vi "IOS_Ephys_WhiskerTracking_Master.vi"() -> ()   [LabVIEW 2013]
uses:
  <vilib>/userdefined/High Color/IMAQdx.ctl
  <vilib>/vision/driver/IMAQdx.llb/IMAQdx Acquisition Mode.ctl
  <vilib>/vision/driver/IMAQdx.llb/IMAQdx Camera Control Mode.ctl
  <vilib>/vision/driver/IMAQdx.llb/IMAQdx Buffer Number Mode.ctl
  <vilib>/DAQmx/read.llb/DAQmx Read (Analog 1D Wfm NChan NSamp).vi
  <vilib>/DAQmx/write.llb/DAQmx Write (Digital 1D Bool NChan 1Samp 1Line).vi
  <vilib>/DAQmx/create/channels.llb/DAQmx Create Channel (DO-Digital Output).vi
  <vilib>/DAQmx/create/channels.llb/DAQmx Create Channel (CO-Pulse Generation-Frequency).vi
  <vilib>/DAQmx/configure/timing.llb/DAQmx Timing (Implicit).vi
  <vilib>/DAQmx/create/channels.llb/DAQmx Create Channel (AI-Voltage-Basic).vi
  <vilib>/DAQmx/configure/timing.llb/DAQmx Timing (Sample Clock).vi
  <vilib>/DAQmx/configure/trigger.llb/DAQmx Start Trigger (Digital Edge).vi
  <vilib>/DAQmx/miscellaneous.llb/DAQmx Fill In Error Info.vi
  <vilib>/vision/driver/NI_Vision_Acquisition_Software.lvlib
panel:
  in  "physical channels":tag="Dev1/ai0:5"
  in  "Whisker Cam ID":T1="cam2"
  in  "WebCam ID":T1="cam1"
  in  "Analog Acquisition Setup":cluster{"Analog Sampling Rate":u16}={"Analog Sampling Rate"=20000} {"Analog Sampling Rate" format="%0.0f"}
  in  "Camera Acquisition Setup":T2={"CBVCam Rate"=30, "WhiskerCam Rate"=150, "WebCam Rate"=15}
  out "Notes Size":i32=7
  out "Notes Reversed":string[](array[string])=["Experimenter", "Animal ID", "Imaged Hemisphere", "Solenoid Pressure", "Isoflurane time", "Session ID", "Amplifier Gain"]
  out "Notes Array":string[](array[string])=["Amplifier Gain", "Session ID", "Isoflurane time", "Solenoid Pressure", "Imaged Hemisphere", "Animal ID", "Experimenter"]
  in  "Session Notes:":T3={"Experimenter"="Experimenter", "Animal ID"="ID", "Imaged Hemisphere"="Hem", "Solenoid Pressure"="psi", "Isoflurane time"="0000", "Session ID"="Test", "Amplifier Gain"="10000"}
  in  "Whisker Cam\nTrigger Source":tag="Dev1/ctr1"
  in  "CBV Cam\nTrigger Source":tag="Dev1/ctr0"
  in  "Left Pad":tag="Dev1/port0/line1"
  in  "Right Pad":tag="Dev1/port0/line0"
  in  "Ctl":tag="Dev1/port0/line3"
  in  "Tail":tag="Dev1/port0/line2"
  in  "Stim \nOffset (s)":dbl=30.0
  in  "Stim \nDuration (s)":dbl=0.1 step=0.1
  in  "Inter-Stim\nInterval (s)":dbl=60.0
  in  "Left Pad":dbl=1.0
  in  "Right Pad":dbl=1.0
  in  "Ctl":dbl=1.0
  in  "Tail":dbl=1.0
  in  "Target Path":path=path "D:/LabVIEW Test Data" caption="Final Saved Location for Files"
  out "Dropped":u32(slide) caption="Dropped Whisker\nCamera Frames" scale=0.0..50.0
  out "Analog file name":string="170302_16_55_2302"
  out "Actual WebCam Frame Rate":dbl(knob)=53292.6 scale=0.0..30.0
  out "WebCam":T4(plugin-control)
  out "Finished Acquiring":bool
  out "Trial Time Elapsed (Min)":cluster{dbl, dbl}(slide)={5.0, 0.09035140000000001} scale=0.0..5.0
  in  "Recording Time (min)":dbl(knob)=5.0 min=0.5 max=10.0 step=0.5 scale=0.0..5.0 scale format="%#_2g"
  in  "Temp Path":path=path "C:/LabView Test Files" caption="Temporary Path for Streamed Data"
  out "Last CBV\nBuffer":i32=162
  in  "Stop":bool
  out "Actual CBVCam\nFrame Rate":dbl(knob)=30.0 scale=0.0..60.0
  out "Last Whisk\nBuffer":u32
  out "Actual WhiskCam\nFrame Rate":dbl(knob) scale=0.0..300.0
  # "File Settings:"
  # "Stimulation Settings:"
  # "Stim. Ratios:"
  # "Output Channels:"
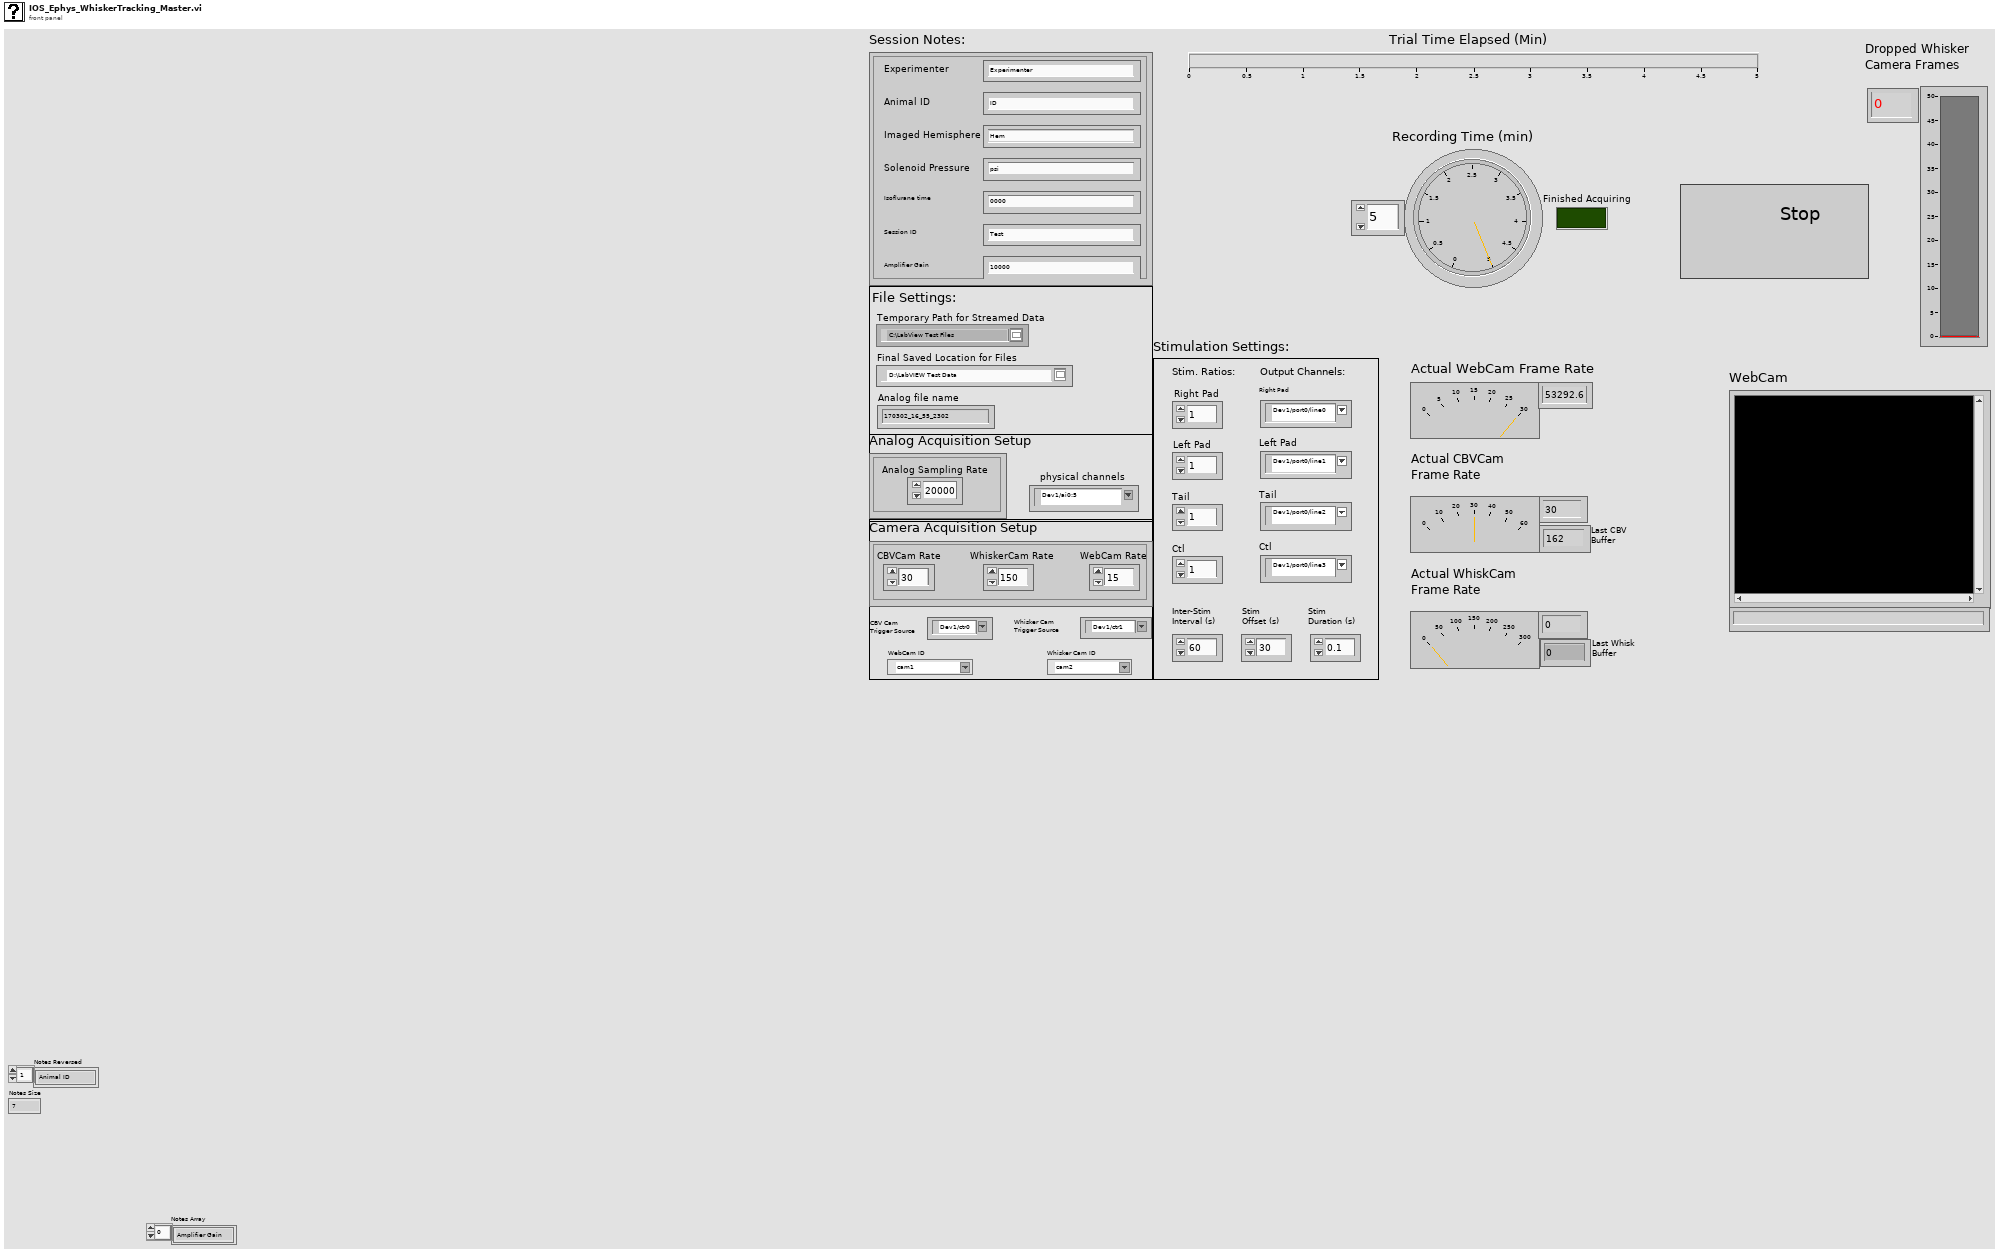
[diagram p1: front panel]
types:
  T1 = typedef "IMAQdx.ctl" = refnum<k21>
  T2 = cluster{"CBVCam Rate":u16, "WhiskerCam Rate":u16, "WebCam Rate":u16}
  T3 = cluster{"Experimenter":string, "Animal ID":string, "Imaged Hemisphere":string, "Solenoid Pressure":string, "Isoflurane time":string, "Session ID":string, "Amplifier Gain":string}
  T4 = typedef "IMAQ Image.ctl" = refnum<image>
  T5 = enum16{"open", "open or create", "create or replace", "create", "open (read-only)"}
  T6 = typedef "Image Type" = u32
  T7 = typedef "NI_Vision_Acquisition_Software.lvlib/IMAQdx Camera Control Mode.ctl" = enum32{"Controller", "Listener"}
  T8 = enum16{"open", "replace", "create", "open or create", "replace or create", "replace or create with confirmation"}
  T9 = typedef "NI_Vision_Acquisition_Software.lvlib/IMAQdx Acquisition Mode.ctl" = enum32{"One Shot", "Continuous"}
  T10 = typedef "IMAQ AVI2 Refnum.ctl" = refnum<k20>
  T11 = enum16{"big-endian, network order", "native, host order", "little-endian"}
  T12 = typedef "NI_Vision_Acquisition_Software.lvlib/IMAQdx Buffer Number Mode.ctl" = enum32{"Next", "Last", "Buffer Number"}
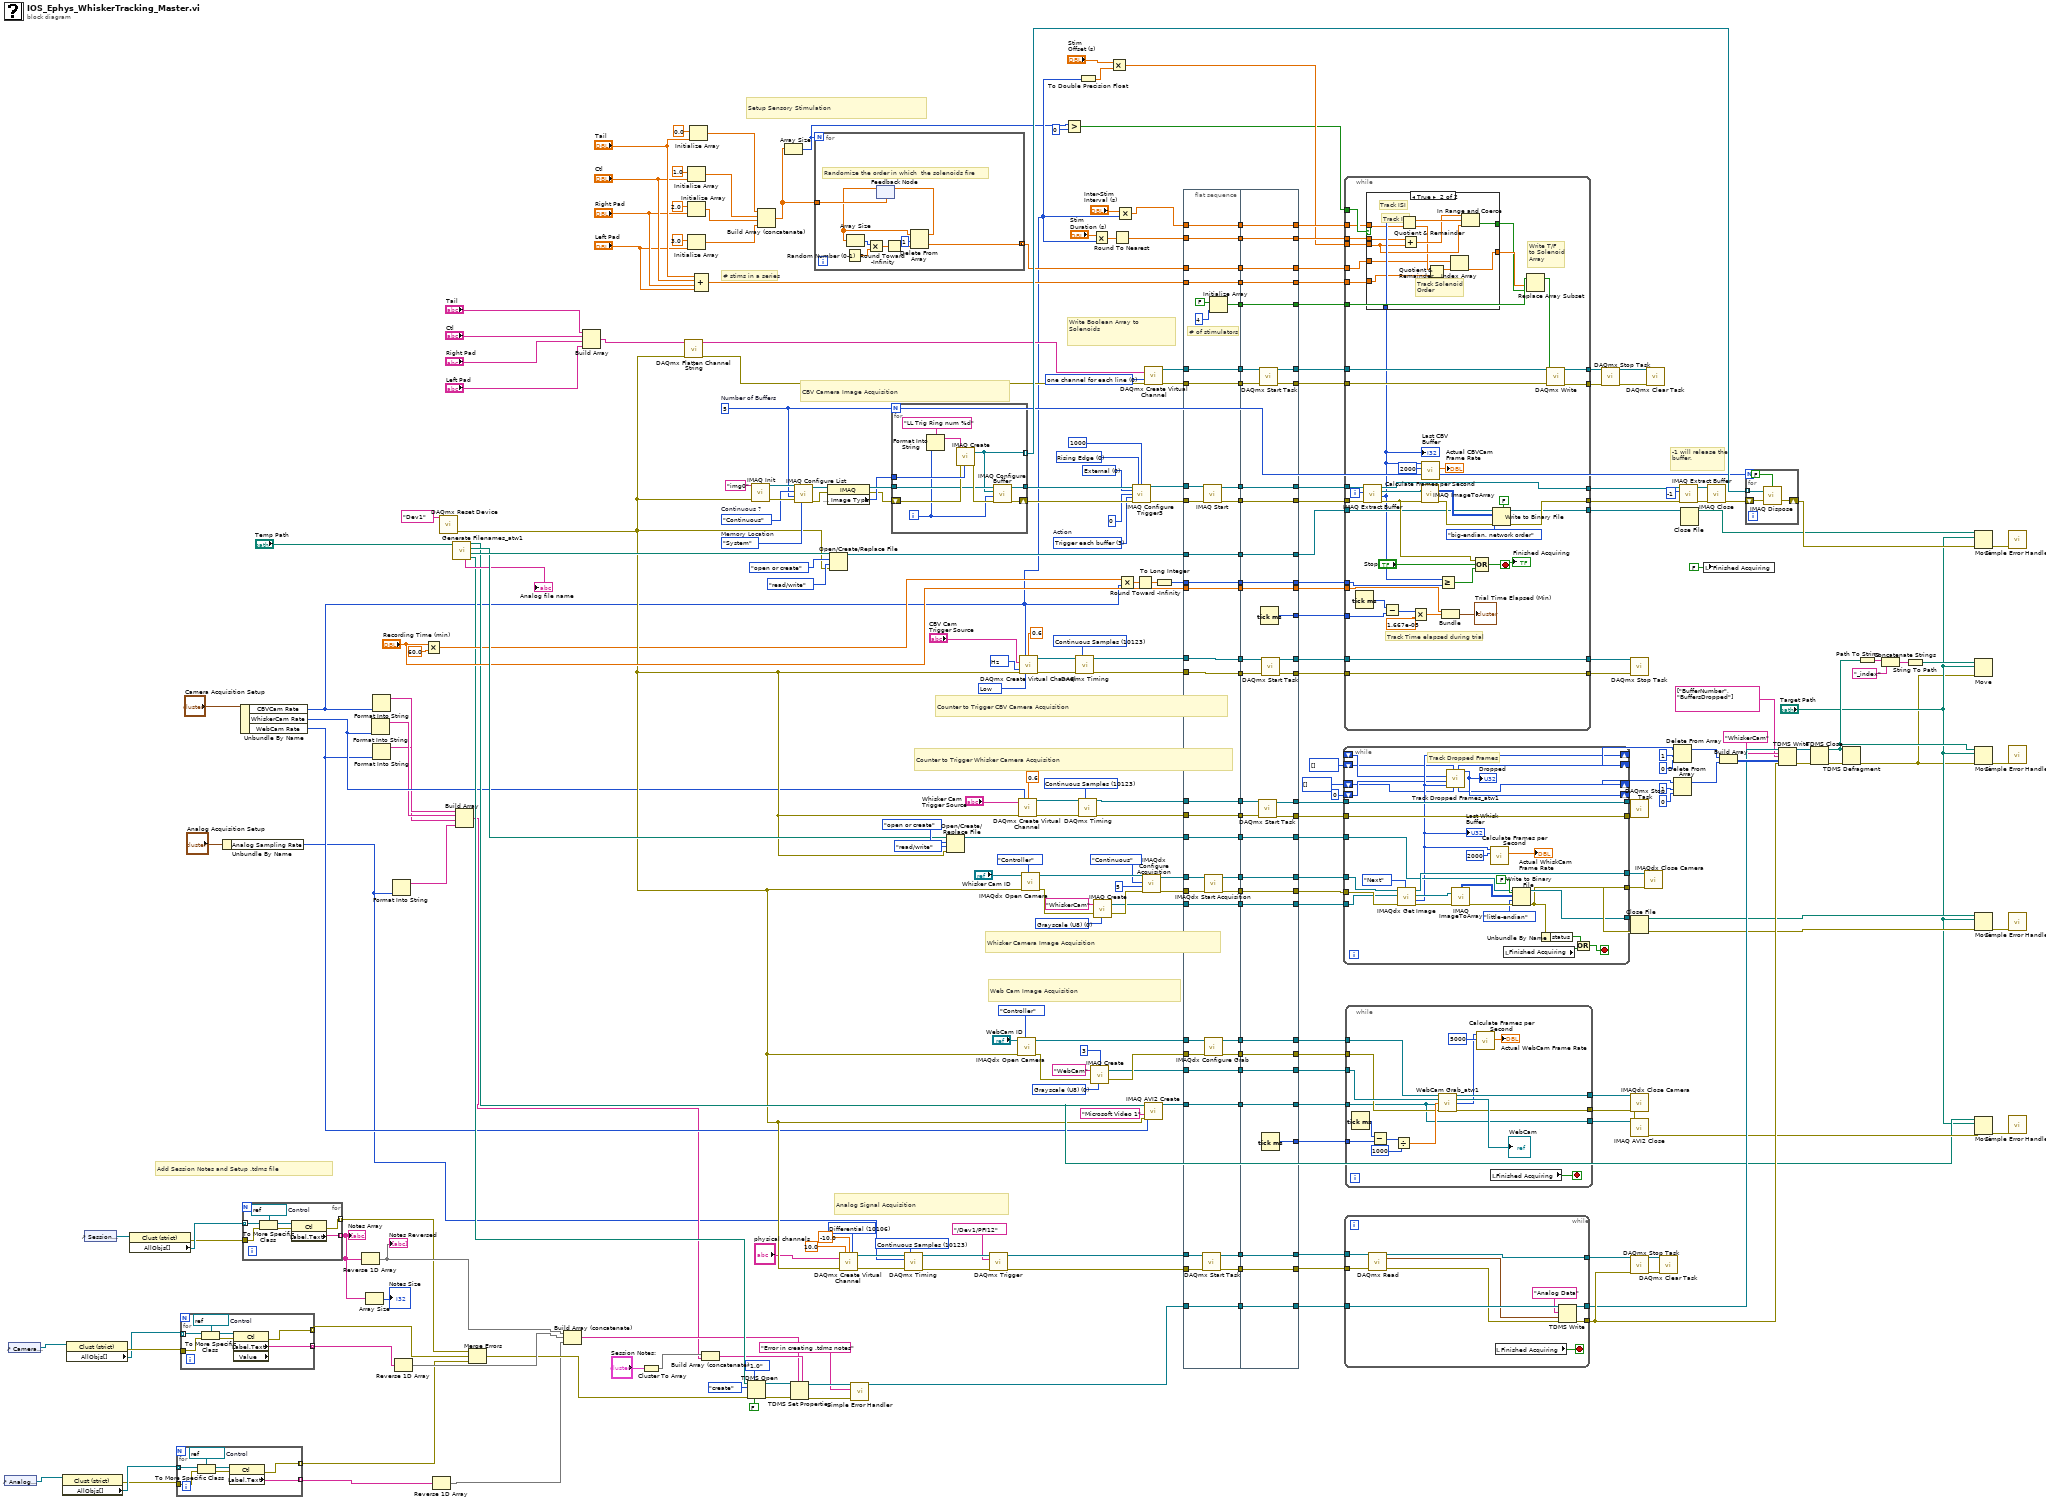
[diagram p0: block diagram]
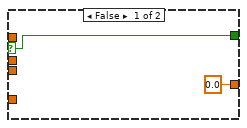
[diagram p2: hidden frame]
diagram:
  w96 = 0 items=["one channel for each line", "one channel for all lines"] ("line grouping")
  w169 = 10123 items=["Finite Samples"=10178, "Continuous Samples"=10123, "Hardware Timed Single Point"=12522] ("sample mode")
  w172 = 10106 items=["default"=-1, "RSE"=10083, "NRSE"=10078, "Differential"=10106, "Pseudodifferential"=12529] ("input terminal configuration")
  w230 = T6 0 items=["Grayscale (U8)", "Grayscale (I16)", "Grayscale (SGL)", "Complex (CSG)", "RGB (U32)", "HSL (U32)", "RGB (U64)", "Grayscale (U16)"] ("Image Type")
  w253 = u32 0 items=["Rising Edge", "Falling Edge"] ("Trigger Polarity")
  w256 = u32 0 items=["External"=0, "RTSI"=1, "ISO In"=2, "Scaled Encoder"=5] ("Trigger Type")
  w246 = 10123 items=["Finite Samples"=10178, "Continuous Samples"=10123, "Hardware Timed Single Point"=12522] ("sample mode")
  w250 = 10373 items=["Hz"=10373] ("units")
  w251 = 10214 items=["High"=10192, "Low"=10214] ("idle state")
  w62 = u32 5  # Number of Buffers
  w254 = u32 3 items=["Disabled", "Trigger start of acquisition", "Trigger start of each buffer list", "Trigger each buffer", "Trigger each line (linescan)", "Trigger end of acquisition"]  # Action
  w261 = enum16{"System", "Onboard"}."System"  # Memory Location
  w260 = enum16{"One-Shot", "Continuous"}."Continuous"  # Continuous ?
  w273 = 10123 items=["Finite Samples"=10178, "Continuous Samples"=10123, "Hardware Timed Single Point"=12522] ("sample mode")
  w280 = T6 0 items=["Grayscale (U8)", "Grayscale (I16)", "Grayscale (SGL)", "Complex (CSG)", "RGB (U32)", "HSL (U32)", "RGB (U64)", "Grayscale (U16)"] ("Image Type")
  # "Setup Sensory Stimulation"
  # "CBV Camera Image Acquisition"
  # "Counter to Trigger CBV Camera Acquisition"
  # "Counter to Trigger Whisker Camera Acquisition"
  # "Whisker Camera Image Acquisition"
  # "Web Cam Image Acquisition"
  # "Add Session Notes and Setup .tdms file"
  # "Analog Signal Acquisition"
  # "Write Boolean Array to \nSolenoids"
  # "# stims in a series"
  # "-1 will release the buffer."
  n1 = control-ref of="Analog Acquisition Setup"() -> (w21:refnum<vi>)
  n2 = control-ref of="Camera Acquisition Setup"() -> (w22:refnum<vi>)
  n3 = property class="Clust (strict)"(reference=w21) -> (error out=w19:errorcluster, "AllObjs[]"=w20:refnum<vi>[])  [unwired: 1 in, 1 out]
  n4 = property class="Clust (strict)"(reference=w22) -> (error out=w45:errorcluster, "AllObjs[]"=w44:refnum<vi>[])  [unwired: 1 in, 1 out]
  n5 = control-ref of="Session Notes:"() -> (w48:refnum<vi>)
  n6 = property class="Clust (strict)"(reference=w48) -> (error out=w51:errorcluster, "AllObjs[]"=w52:refnum<vi>[])  [unwired: 1 in, 1 out]
  n7 = for {
    tunnel: [w292] -> w17 mode=indexing
    tunnel: w20 -> [w291] mode=indexing
    tunnel: w19 -> [w290]
    tunnel: [w288] -> w18 mode=indexing
    w293 = refnum<vi> refnum  # Control
    n8 = To More Specific Class(target class=w293, reference=w291, error in=w290) -> (specific class reference=w294:refnum<vi>, error out=w289:errorcluster)
    n9 = property class="Ctl"(reference=w294, error in=w289) -> (error out=w288:errorcluster, "Label.Text"=w292:string)  [unwired: 1 out]
  }
  n10 = for {
    tunnel: [w299] -> w46 mode=indexing
    tunnel: w44 -> [w298] mode=indexing
    tunnel: w45 -> [w297]
    tunnel: [w295] -> w28 mode=indexing
    w300 = refnum<vi> refnum  # Control
    n11 = To More Specific Class(target class=w300, reference=w298, error in=w297) -> (specific class reference=w301:refnum<vi>, error out=w296:errorcluster)
    n12 = property class="Ctl" props=["Label", "Text", "Value"](reference=w301, error in=w296) -> (error out=w295:errorcluster, "Label.Text"=w299:string)  [unwired: 2 out]
  }
  n13 = Unbundle By Name("Analog Acquisition Setup") -> ("Analog Sampling Rate"=w4:u16)
  n14 = Unbundle By Name("Camera Acquisition Setup") -> ("CBVCam Rate"=w13:u16, "WhiskerCam Rate"=w12:u16, "WebCam Rate"=w11:u16)
  n15 = for {
    tunnel: [w306] -> w50 mode=indexing
    tunnel: w52 -> [w305] mode=indexing
    tunnel: w51 -> [w304]
    tunnel: [w302] -> w29 mode=indexing
    w307 = refnum<vi> refnum  # Control
    n16 = To More Specific Class(target class=w307, reference=w305, error in=w304) -> (specific class reference=w308:refnum<vi>, error out=w303:errorcluster)
    n17 = property class="Ctl"(reference=w308, error in=w303) -> (error out=w302:errorcluster, "Label.Text"=w306:string)  [unwired: 1 out]
  }
  "Notes Array" <- w50
  n18 = Reverse 1D Array(array=w50) -> (reversed array=w34:string[])
  "Notes Reversed" <- w34
  n19 = Array Size(array=w50) -> (size(s)=→"Notes Size":i32)
  n20 = Format Into String(w12) -> (resulting string=w9:string)  [unwired: 3 in, 1 out]
  n21 = Format Into String(w13) -> (resulting string=w10:string)  [unwired: 3 in, 1 out]
  n22 = Format Into String(w11) -> (resulting string=w8:string)  [unwired: 3 in, 1 out]
  n23 = Format Into String(w4) -> (resulting string=w7:string)  [unwired: 3 in, 1 out]
  n24 = Reverse 1D Array(array=w46) -> (reversed array=w33:string[])
  n25 = Multiply(x="Recording Time (min)", y=60.0) -> (x*y=w43:dbl)
  n26 = Reverse 1D Array(array=w17) -> (reversed array=w16:string[])
  n27 = call <vilib>:"DAQmx Reset Device.vi"("device in"=tag "Dev1") -> ("error out"=w47:errorcluster)  [unwired: 14 in]
  n28 = call "Generate Filenames_atw1.vi"("path"="Temp Path") -> ("TDMS Path"=w40:path, "Dalsa Path"=w238:path, "Basler Path"=w233:path, "WebCam Path"=w124:path, "Analog file name"=→"Analog file name":string)  [unwired: 5 in, 1 out]
  n29 = Build Array(w10, w9, w8, w7) -> (w6:string[])
  n30 = Merge Errors(w29, w28, w18) -> (w27:errorcluster)
  n31 = Build Array (concatenate)(w34, w33, w16) -> (w31:string[])
  n32 = Build Array("Tail", "Ctl", "Right Pad", "Left Pad") -> (w54:tag[])
  n33 = Cluster To Array(cluster="Session Notes:") -> (array=w41:string[])
  n34 = call <vilib>:"DAQmx Flatten Channel String.vi"("names in"=w54, "error in"=w47) -> ("names out"=w59:string, "error out"=w53:errorcluster)  [unwired: 12 in]
  n35 = Initialize Array(2.0 ("element"), "Right Pad") -> (w105:dbl[])
  n36 = Initialize Array(3.0 ("element"), "Left Pad") -> (w104:dbl[])
  n37 = Initialize Array(1.0 ("element"), "Ctl") -> (w106:dbl[])
  n38 = Initialize Array(0.0 ("element"), "Tail") -> (w107:dbl[])
  n39 = Compound Arithmetic op=ADD("Tail", "Ctl", "Right Pad", "Left Pad") -> (w80:dbl)
  n40 = Build Array (concatenate)(w41, w6) -> (w32:string[])
  n41 = TDMS Open(6:FALSE ("disable buffering? (T)"), 7:enum16{"1.0", "2.0"}."1.0" ("file format version (2.0)"), 8:w27, 10:T5."create" ("operation (0:open)"), 11:w40) -> (0:w35:errorcluster, 3:w36:refnum<k34>)  [unwired: 2 in]
  n42 = call <vilib>:"IMAQ Init.vi"("error in (no error)"=w47, "Interface Name"="img0") -> ("error out"=w271:errorcluster, "IMAQ Session Out"=w272:refnum<k11>)  [unwired: 8 out]
  n43 = Build Array (concatenate)(w107, w106, w105, w104) -> (w99:dbl[])
  n44 = Array Size(array=w99) -> (size(s)=w3:i32)
  n45 = TDMS Set Properties(5:w32, 7:w31, 8:w35, 11:w36) -> (0:w26:errorcluster, 3:w30:refnum<k34>)  [unwired: 2 in, 2 out]
  n46 = call <vilib>:"IMAQ Configure List.vi"("Memory Location"=w261, "error in (no error)"=w271, "Number of buffers"=w62, "Continuous?"=w260, "IMAQ Session In"=w272) -> ("error out"=w269:errorcluster, "IMAQ Session Out"=w268:refnum<k11>)  [unwired: 1 in, 4 out]
  n47 = for {
    N: w3 -> [_]
    tunnel: w99 -> [w312]
    tunnel: [w309] -> w77 mode=concatenating
    # "Randomize the order in which  the solenoids fire"
    n48 = Random Number (0-1)() -> (number: 0 to 1=w316:dbl)
    n49 = feedback #1(w312) -> (w311:dbl[])
    n50 = Array Size(array=w311) -> (size(s)=w317:i32)
    n51 = Multiply(x=w317, y=w316) -> (x*y=w315:dbl)
    n52 = Round Toward -Infinity(1:w315) -> (0:w314:dbl)
    n53 = Delete From Array(array=w311, length=1, index=w314) -> (deleted portion=w309:dbl[], array with subset deleted=w310:dbl[])
    n54 = feedback-in #1(w310) -> ()
  }
  n55 = property class="IMAQ"(reference=w268, error in=w269) -> (reference out=w264:refnum<k11>, error out=w262:errorcluster, "Image Parameters : Image Type"=w263:u32)
  n56 = Open/Create/Replace File(file path (use dialog)=w238, error in=w47, operation (0:open)=T8."open or create", access (0:read/write)=enum16{"read/write", "read-only", "write-only"}."read/write") -> (refnum out=w173:refnum<file>)  [unwired: 2 in, 2 out]
  n57 = call-poly <vilib>:"DAQmx Create Virtual Channel.vi"("maximum value"=10.0, "minimum value"=-10.0, "input terminal configuration"=w172, "physical channels"="physical channels", "error in"=w47) -> ("task out"=w171:refnum<k21>, "error out"=w170:errorcluster)  [unwired: 9 in]
  n58 = call <vilib>:"Simple Error Handler.vi"("error source (\" \")"="Error in creating .tdms notes" ("error source (\" \")"), "error in (no error)"=w26) -> ()  [unwired: 3 in, 5 out]
  n59 = for {
    N: w62 -> [_]
    tunnel: [w327] -> w258
    tunnel: w263 -> [w325]
    tunnel: w264 -> [w322]
    shift-right: [w326] -> w257
    shift-left: w262 -> [w324]
    tunnel: [w318] -> w259 mode=indexing
    i -> [w319]
    n60 = Format Into String(format string="LL Trig Ring num %d", w319) -> (resulting string=w321:string)  [unwired: 2 in, 1 out]
    n61 = call "IMAQ Create"("Image Name"=w321, "Image Type"=w325, "error in (no error)"=w324) -> ("New Image"=w318:T4, "error out"=w323:errorcluster)  [unwired: 1 in, 1 out]
    n62 = call <vilib>:"IMAQ Configure Buffer.vi"("error in (no error)"=w323, "Buffer Number"=w319, "Image In"=w318, "IMAQ Session In"=w322) -> ("error out"=w326:errorcluster, "IMAQ Session Out"=w327:refnum<k11>)  [unwired: 2 in, 4 out]
  }
  n63 = call-poly <vilib>:"DAQmx Timing.vi"("task/channels in"=w171, "sample mode"=w169, "rate"=w4, "error in"=w170) -> ("task out"=w168:refnum<k21>, "error out"=w167:errorcluster)  [unwired: 10 in]
  n64 = Open/Create/Replace File(file path (use dialog)=w233, error in=w47, operation (0:open)=T8."open or create", access (0:read/write)=enum16{"read/write", "read-only", "write-only"}."read/write") -> (refnum out=w193:refnum<file>)  [unwired: 2 in, 2 out]
  n65 = call-poly <vilib>:"DAQmx Trigger.vi"("task/channels in"=w168, "source"=tag "/Dev1/PFI12", "error in"=w167) -> ("task out"=w165:refnum<k21>, "error out"=w164:errorcluster)  [unwired: 11 in]
  n66 = call <vilib>:"IMAQdx Open Camera.vi"("Camera Control Mode"=IMAQdx_Camera_Control_Mode."Controller", "error in"=w47, "Session In"="WebCam ID") -> ("error out"=w225:errorcluster, "Session Out"=w223:T1)  [unwired: 7 in]
  n67 = call-poly <vilib>:"DAQmx Create Virtual Channel.vi"("frequency"=w12, "duty cycle"=0.6, "counter"="Whisker Cam\nTrigger Source", "error in"=w47) -> ("task out"=w275:refnum<k21>, "error out"=w274:errorcluster)  [unwired: 10 in]
  n68 = call-poly <vilib>:"DAQmx Create Virtual Channel.vi"("frequency"=w13, "duty cycle"=0.6, "counter"="CBV Cam\nTrigger Source", "units"=w250, "error in"=w47, "idle state"=w251) -> ("task out"=w248:refnum<k21>, "error out"=w247:errorcluster)  [unwired: 8 in]
  n69 = call <vilib>:"IMAQdx Open Camera.vi"("Camera Control Mode"=IMAQdx_Camera_Control_Mode."Controller", "error in"=w47, "Session In"="Whisker Cam ID") -> ("error out"=w283:errorcluster, "Session Out"=w286:T1)  [unwired: 7 in]
  n70 = Greater?(x=w3, y=0) -> (0:w1:bool)
  n71 = call-poly <vilib>:"DAQmx Timing.vi"("task/channels in"=w248, "sample mode"=w246, "error in"=w247) -> ("task out"=w155:refnum<k21>, "error out"=w153:errorcluster)  [unwired: 11 in]
  n72 = call-poly <vilib>:"DAQmx Timing.vi"("task/channels in"=w275, "sample mode"=w273, "error in"=w274) -> ("task out"=w151:refnum<k21>, "error out"=w149:errorcluster)  [unwired: 11 in]
  n73 = To Double Precision Float(number=w13) -> (double precision float=w60:dbl)
  n74 = call "IMAQ Create"("Border Size"=3, "Image Name"="WebCam", "Image Type"=w230, "error in (no error)"=w225) -> ("New Image"=w222:T4, "error out"=w224:errorcluster)  [unwired: 1 in]
  n75 = Multiply(x="Stim \nDuration (s)", y=w13) -> (x*y=w71:dbl)
  n76 = call "IMAQ Create"("Image Name"="WhiskerCam", "Image Type"=w280, "error in (no error)"=w283) -> ("New Image"=w196:T4, "error out"=w281:errorcluster)  [unwired: 2 in]
  n77 = Multiply(x="Stim \nOffset (s)", y=w60) -> (x*y=w61:dbl)
  n78 = Round To Nearest(number=w71) -> (nearest integer value=w70:dbl)
  n79 = Multiply(x="Inter-Stim\nInterval (s)", y=w13) -> (x*y=w84:dbl)
  n80 = Multiply(x=w43, y=w13) -> (x*y=w235:dbl)
  n81 = call <vilib>:"IMAQ Configure Trigger3.vi"("IMAQ Session In"=w258, "Polarity"=w253, "Frame timeout (ms)"=u32 1000 ("Frame Timeout (ms)"), "Type"=w256, "Line Number"=u32 0 ("Trigger Line Number"), "Action"=w254, "error in (no error)"=w257) -> ("IMAQ Session Out"=w192:refnum<k11>, "error out"=w191:errorcluster)  [unwired: 2 in, 5 out]
  n82 = Round Toward -Infinity(1:w235) -> (0:w234:dbl)
  n83 = call <vilib>:"IMAQdx Configure Acquisition.vi"("error in"=w281, "Number of Buffers"=u32 5, "Continuous?"=IMAQdx_Acquisition_Mode."Continuous", "Session In"=w286) -> ("error out"=w203:errorcluster, "Session Out"=w204:T1)  [unwired: 6 in]
  n84 = call "IMAQ AVI2 Create"("error in (no error)"=w47, "Codec"="Microsoft Video 1", "Frames Per Second"=w11, "AVI Path"=w124) -> ("AVI Refnum"=w215:T10)  [unwired: 6 in, 1 out]
  n85 = call-poly <vilib>:"DAQmx Create Virtual Channel.vi"("lines"=w59, "line grouping"=w96, "error in"=w53) -> ("task out"=w94:refnum<k21>, "error out"=w92:errorcluster)  [unwired: 11 in]
  n86 = To Long Integer(number=w234) -> (32bit integer=w181:i32)
  n87 = flat-sequence {
    tunnel: w224 -> [w364]
    tunnel: w223 -> [w363]
    tunnel: w222 -> [w362]
    tunnel: [w362] -> w221
    tunnel: [w361] -> w219
    tunnel: [w360] -> w217
    tunnel: w215 -> [w359]
    tunnel: [w359] -> w214
    tunnel: w204 -> [w358]
    tunnel: w203 -> [w357]
    tunnel: [w356] -> w201
    tunnel: [w355] -> w199
    tunnel: [w354] -> w197
    tunnel: w196 -> [w354]
    tunnel: [w353] -> w194
    tunnel: w193 -> [w353]
    tunnel: w192 -> [w352]
    tunnel: w191 -> [w351]
    tunnel: [w350] -> w189
    tunnel: [w349] -> w187
    tunnel: w181 -> [w348]
    tunnel: [w348] -> w180
    tunnel: "Recording Time (min)" -> [w347]
    tunnel: [w347] -> w177
    tunnel: [w346] -> w174
    tunnel: w173 -> [w346]
    tunnel: w165 -> [w345]
    tunnel: w164 -> [w344]
    tunnel: [w343] -> w163
    tunnel: [w342] -> w162
    tunnel: [w341] -> w157
    tunnel: w30 -> [w341]
    tunnel: w155 -> [w340]
    tunnel: [w340] -> w154
    tunnel: w153 -> [w339]
    tunnel: [w339] -> w152
    tunnel: w151 -> [w338]
    tunnel: [w338] -> w150
    tunnel: w149 -> [w337]
    tunnel: [w337] -> w148
    tunnel: w94 -> [w336]
    tunnel: [w336] -> w95
    tunnel: w92 -> [w335]
    tunnel: [w335] -> w93
    tunnel: w84 -> [w334]
    tunnel: [w334] -> w83
    tunnel: [w333] -> w81
    tunnel: w70 -> [w333]
    tunnel: w80 -> [w332]
    tunnel: [w332] -> w79
    tunnel: w77 -> [w331]
    tunnel: [w331] -> w76
    tunnel: [w329] -> w74
    tunnel: [w399] -> w226
    tunnel: w221 -> [w398]
    tunnel: [w398] -> w220
    tunnel: w219 -> [w397]
    tunnel: [w397] -> w218
    tunnel: w217 -> [w396]
    tunnel: [w396] -> w216
    tunnel: w214 -> [w395]
    tunnel: [w395] -> w213
    tunnel: [w377] -> w209
    tunnel: [w376] -> w207
    tunnel: [w394] -> w202
    tunnel: w201 -> [w394]
    tunnel: [w393] -> w200
    tunnel: w199 -> [w393]
    tunnel: [w392] -> w198
    tunnel: w197 -> [w392]
    tunnel: [w391] -> w195
    tunnel: w194 -> [w391]
    tunnel: [w390] -> w190
    tunnel: w189 -> [w390]
    tunnel: [w389] -> w188
    tunnel: w187 -> [w389]
    tunnel: [w381] -> w185
    tunnel: [w380] -> w183
    tunnel: [w388] -> w182
    tunnel: w180 -> [w387]
    tunnel: [w387] -> w179
    tunnel: [w386] -> w178
    tunnel: w177 -> [w386]
    tunnel: [w385] -> w175
    tunnel: w174 -> [w385]
    tunnel: [w384] -> w160
    tunnel: w163 -> [w384]
    tunnel: [w383] -> w161
    tunnel: w162 -> [w383]
    tunnel: [w382] -> w158
    tunnel: w157 -> [w382]
    tunnel: w154 -> [w379]
    tunnel: w152 -> [w378]
    tunnel: w150 -> [w375]
    tunnel: w148 -> [w374]
    tunnel: w95 -> [w373]
    tunnel: w93 -> [w372]
    tunnel: [w371] -> w91
    tunnel: [w370] -> w90
    tunnel: [w369] -> w85
    tunnel: w83 -> [w369]
    tunnel: [w368] -> w82
    tunnel: w81 -> [w368]
    tunnel: w79 -> [w367]
    tunnel: [w367] -> w78
    tunnel: w76 -> [w366]
    tunnel: [w366] -> w75
    tunnel: w74 -> [w365]
    tunnel: [w365] -> w73
    frame #0 {
      # "# of stimulators"
      n88 = call <vilib>:"DAQmx Start Task.vi"("task/channels in"=w345, "error in"=w344) -> ("task out"=w343:refnum<k21>, "error out"=w342:errorcluster)  [unwired: 12 in]
      n89 = call <vilib>:"IMAQ Start.vi"("error in (no error)"=w351, "IMAQ Session In"=w352) -> ("error out"=w349:errorcluster, "IMAQ Session Out"=w350:refnum<k11>)  [unwired: 8 out]
      n90 = call <vilib>:"IMAQdx Configure Grab.vi"("error in"=w364, "Session In"=w363) -> ("error out"=w360:errorcluster, "Session Out"=w361:T1)  [unwired: 8 in]
      n91 = call <vilib>:"IMAQdx Start Acquisition.vi"("error in"=w357, "Session In"=w358) -> ("error out"=w355:errorcluster, "Session Out"=w356:T1)  [unwired: 8 in]
      n92 = Initialize Array(FALSE, 4 ("dimension size")) -> (w329:bool[])
    }
    frame #1 {
      n93 = call <vilib>:"DAQmx Start Task.vi"("task/channels in"=w375, "error in"=w374) -> ("task out"=w377:refnum<k21>, "error out"=w376:errorcluster)  [unwired: 12 in]
      n94 = call <vilib>:"DAQmx Start Task.vi"("task/channels in"=w373, "error in"=w372) -> ("task out"=w371:refnum<k21>, "error out"=w370:errorcluster)  [unwired: 12 in]
      n95 = Tick Count (ms)() -> (millisecond timer value=w388:u32)
      n96 = call <vilib>:"DAQmx Start Task.vi"("task/channels in"=w379, "error in"=w378) -> ("task out"=w381:refnum<k21>, "error out"=w380:errorcluster)  [unwired: 12 in]
      n97 = Tick Count (ms)() -> (millisecond timer value=w399:u32)
    }
  }
  n98 = while {
    tunnel: w209 -> [w418]
    tunnel: [w419] -> w208
    tunnel: w207 -> [w419]
    tunnel: [w418] -> w206
    tunnel: [w417] -> w64
    tunnel: [w401] -> w63
    tunnel: [w416] -> w205
    tunnel: w202 -> [w415]
    tunnel: w200 -> [w414]
    tunnel: w198 -> [w413]
    tunnel: w195 -> [w412]
    shift-right: [w411] -> _
    shift-left: _ -> [w410]
    shift-right: [w409] -> _
    shift-left: u32 0 ("New Lost") -> [w408]
    shift-right: [w407] -> w144
    shift-left: u32[] [] ("NewBuffNum") -> [w406]
    shift-right: [w405] -> w141
    shift-left: u32[] [] ("NewNumLost") -> [w404]
    stop <- w403 stop-if-true
    # "Track Dropped Frames"
    n99 = call <vilib>:"IMAQdx Get Image.vi"("Buffer Number Mode (Next)"=IMAQdx_Buffer_Number_Mode."Next", "error in"=w414, "Image In"=w413, "Session In"=w415) -> ("error out"=w427:errorcluster, "Buffer Number Out"=w411:u32, "Image Out"=w426:T4, "Session Out"=w417:T1)  [unwired: 4 in]
    "Last Whisk\nBuffer" <- w411
    n100 = call "Track Dropped Frames_atw1.vi"("NumLost"=w404, "BuffNum"=w406, "Curr Buffer"=w411, "Prev Lost"=w408, "Prev Buffer"=w410) -> ("New Lost"=w409:u32, "NewNumLost"=w405:u32[], "NewBuffNum"=w407:u32[])  [unwired: 4 in]
    "Dropped" <- w409
    n101 = call "IMAQ ImageToArray"("error in (no error)"=w427, "Image"=w426) -> ("error out"=w425:errorcluster, "Image Pixels (U8)"=w424:u8[][])  [unwired: 2 in, 3 out]
    n102 = call <vilib>:"Calculate Frames per Second.vi"("Update Interval (ms)"=u32 2000, "Buffer Number"=w411) -> ("Processed Frames/s"=→"Actual WhiskCam\nFrame Rate":dbl)  [unwired: 7 in, 2 out]
    n103 = local read "Finished Acquiring"() -> (w402:bool)
    n104 = Write to Binary File(file (use dialog)=w412, data=w424, error in=w425, 5:FALSE ("prepend array or string size? (T)"), 9:T11."little-endian" ("byte order (0:big-endian, network order)")) -> (refnum out=w416:refnum<file>, error out=w401:errorcluster)  [unwired: 1 in, 1 out]
    n105 = Unbundle By Name(w401) -> ("status"=w400:bool)
    n106 = Or(x=w400, y=w402) -> (x .or. y?=w403:bool)
  }
  n107 = while {
    tunnel: w190 -> [w470]
    tunnel: w188 -> [w471]
    tunnel: [w463] -> w240
    tunnel: [w461] -> w241
    tunnel: [w460] -> w239
    tunnel: [w452] -> w186
    tunnel: w185 -> [w452]
    tunnel: [w451] -> w184
    tunnel: w183 -> [w451]
    tunnel: w182 -> [w450]
    tunnel: w179 -> [w449]
    tunnel: w178 -> [w448]
    tunnel: w175 -> [w446]
    tunnel: w91 -> [w444]
    tunnel: w90 -> [w443]
    tunnel: [w442] -> w89
    tunnel: [w441] -> w88
    tunnel: w85 -> [w435]
    tunnel: w82 -> [w434]
    tunnel: w78 -> [w432]
    tunnel: w75 -> [w430]
    tunnel: w73 -> [w440]
    tunnel: w61 -> [w433]
    tunnel: w1 -> [w437]
    i -> [w469]
    stop <- w453 stop-if-true
    # "Track Time elapsed during trial"
    # "Write T/F \nto Solenoid\nArray"
    # "Track ISI"
    n108 = Tick Count (ms)() -> (millisecond timer value=w457:u32)
    n109 = call <vilib>:"IMAQ Extract Buffer.vi"("error in (no error)"=w471, "Buffer to extract"=w469, "IMAQ Session In"=w470) -> ("error out"=w458:errorcluster, "Buffer Number"=w436:i32, "Image Out"=w467:T4, "IMAQ Session Out"=w461:refnum<k11>)  [unwired: 5 out]
    "Last CBV\nBuffer" <- w436
    n110 = case shown="True" w437 {
      selector: w437 -> [w473 _]
      tunnel: w436 -> [_ w483]
      tunnel: w435 -> [_ w482]
      tunnel: w434 -> [_ w481]
      tunnel: w433 -> [_ w480]
      tunnel: w432 -> [_ w477]
      tunnel: [0.0 ("element") w474] -> w431
      tunnel: w430 -> [_ w476]
      tunnel: [w473 w475] -> w429
      frame False {
      }
      frame True {
        # "Track Solenoid\nOrder"
        # "Track ISI"
        n111 = Quotient & Remainder(x=w483, y=w482) -> (x-y*floor(x/y)=w485:dbl, floor(x/y)=w478:dbl)
        n112 = Add(x=w481, y=w480) -> (x+y=w484:dbl)
        n113 = Quotient & Remainder(x=w478, y=w477) -> (x-y*floor(x/y)=w479:dbl)  [unwired: 1 out]
        n114 = Index Array(array=w476, index=w479) -> (element=w474:dbl)
        n115 = In Range and Coerce(upper limit=w484, x=w485, lower limit=w480) -> (In Range?=w475:bool)  [unwired: 1 out]
      }
    }
    n116 = Subtract(x=w457, y=w450) -> (x-y=w456:u32)
    n117 = Multiply(x=w456, y=1.667e-05) -> (x*y=w455:dbl)
    n118 = call "IMAQ ImageToArray"("error in (no error)"=w458, "Image"=w467) -> ("error out"=w466:errorcluster, "Image Pixels (I16)"=w465:i16[][])  [unwired: 2 in, 3 out]
    n119 = call <vilib>:"Calculate Frames per Second.vi"("Update Interval (ms)"=u32 2000, "Buffer Number"=w436) -> ("Processed Frames/s"=→"Actual CBVCam\nFrame Rate":dbl)  [unwired: 7 in, 2 out]
    n120 = Greater Or Equal?(x=w436, y=w449) -> (x >= y?=w454:bool)
    n121 = Bundle("Recording Time (min)"=w448, w455) -> (→"Trial Time Elapsed (Min)":cluster{"Recording Time (min)":dbl, dbl})  [unwired: 1 in]
    n122 = Compound Arithmetic op=OR(w458, "Stop", w454) -> (w453:bool)
    "Finished Acquiring" <- w453
    n123 = Write to Binary File(file (use dialog)=w446, data=w465, error in=w466, 5:FALSE ("prepend array or string size? (T)"), 9:T11."big-endian, network order" ("byte order (0:big-endian, network order)")) -> (refnum out=w460:refnum<file>, error out=w463:errorcluster)  [unwired: 1 in, 1 out]
    n124 = Replace Array Subset(array=w440, new element=w429, index=w431) -> (w439:bool[])
    n125 = call-poly <vilib>:"DAQmx Write.vi"("task/channels in"=w444, "data"=w439, "error in"=w443) -> ("task out"=w442:refnum<k21>, "error out"=w441:errorcluster)  [unwired: 10 in, 1 out]
  }
  n126 = while {
    tunnel: w161 -> [w495]
    tunnel: w160 -> [w494]
    tunnel: w158 -> [w493]
    tunnel: [w492] -> w134
    tunnel: [w491] -> w135
    tunnel: [w490] -> w156
    stop <- w489 stop-if-true
    n127 = call-poly <vilib>:"DAQmx Read.vi"("task/channels in"=w494, "error in"=w495) -> ("task out"=w490:refnum<k21>, "data"=w486:waveform(dbl)[], "error out"=w487:errorcluster)  [unwired: 11 in]
    n128 = local read "Finished Acquiring"() -> (w489:bool)
    n129 = TDMS Write(0:w493, 5:"Analog Data" ("group name in (Untitled)"), 9:w486, 11:w487) -> (4:w492:refnum<k34>, 15:w491:errorcluster)  [unwired: 2 in, 2 out]
  }
  n130 = while {
    tunnel: w226 -> [w505]
    tunnel: w220 -> [w503]
    tunnel: w218 -> [w502]
    tunnel: w216 -> [w501]
    tunnel: w213 -> [w497]
    tunnel: [w499] -> w212
    tunnel: [w498] -> w210
    tunnel: [w497] -> w211
    stop <- w508 stop-if-true
    n131 = Tick Count (ms)() -> (millisecond timer value=w509:u32)
    n132 = Subtract(x=w509, y=w505) -> (x-y=w510:u32)
    n133 = Divide(x=w510, y=u32 1000) -> (x/y=w504:dbl)
    n134 = call "WebCam Grab_atw1.vi"("Session In"=w502, "Image In"=w503, "Trial Time"=w504, "AVI Refnum"=w497, "error in"=w501) -> ("Session Out"=w499:T1, "WebCam Img Out"=→"WebCam":T4, "Buffer Number Out"=w496:u32, "error out"=w498:errorcluster)  [unwired: 7 in]
    n135 = call <vilib>:"Calculate Frames per Second.vi"("Update Interval (ms)"=u32 5000, "Buffer Number"=w496) -> ("Processed Frames/s"=→"Actual WebCam Frame Rate":dbl)  [unwired: 7 in, 2 out]
    n136 = local read "Finished Acquiring"() -> (w508:bool)
  }
  n137 = call <vilib>:"DAQmx Stop Task.vi"("task/channels in"=w89, "error in"=w88) -> ("task out"=w87:refnum<k21>, "error out"=w86:errorcluster)  [unwired: 12 in]
  n138 = call <vilib>:"DAQmx Stop Task.vi"("task/channels in"=w186, "error in"=w184) -> ()  [unwired: 12 in, 2 out]
  n139 = call <vilib>:"DAQmx Stop Task.vi"("task/channels in"=w206, "error in"=w208) -> ()  [unwired: 12 in, 2 out]
  n140 = Close File(refnum=w205, error in=w63) -> (path=w123:path, error out=w122:errorcluster)
  n141 = call <vilib>:"IMAQdx Close Camera.vi"("error in"=w210, "Session In"=w212) -> ()  [unwired: 9 in, 1 out]
  n142 = call "IMAQ AVI2 Close"("error in (no error)"=w210, "AVI Refnum"=w211) -> ("error out"=w125:errorcluster)  [unwired: 9 in]
  n143 = call <vilib>:"DAQmx Stop Task.vi"("task/channels in"=w156, "error in"=w135) -> ("task out"=w66:refnum<k21>, "error out"=w65:errorcluster)  [unwired: 12 in]
  n144 = call <vilib>:"IMAQdx Close Camera.vi"("error in"=w63, "Session In"=w64) -> ()  [unwired: 9 in, 1 out]
  n145 = call <vilib>:"DAQmx Clear Task.vi"("task in"=w87, "error in"=w86) -> ()  [unwired: 13 in, 1 out]
  n146 = call <vilib>:"DAQmx Clear Task.vi"("task in"=w66, "error in"=w65) -> ()  [unwired: 13 in, 1 out]
  n147 = Delete From Array(array=w144, length=1, index=0) -> (array with subset deleted=w138:u32[])  [unwired: 1 out]
  n148 = Delete From Array(array=w141, length=1, index=0) -> (array with subset deleted=w137:u32[])  [unwired: 1 out]
  n149 = call <vilib>:"IMAQ Extract Buffer.vi"("error in (no error)"=w240, "Buffer to extract"=-1, "IMAQ Session In"=w241) -> ("error out"=w266:errorcluster, "IMAQ Session Out"=w265:refnum<k11>)  [unwired: 7 out]
  n150 = Close File(refnum=w239) -> (path=w126:path)  [unwired: 1 in, 1 out]
  n151 = local write "Finished Acquiring"(FALSE ("Finished Acquiring")) -> ()
  n152 = call <vilib>:"IMAQ Close.vi"("error in (no error)"=w266, "IMAQ Session In"=w265) -> ("error out"=w270:errorcluster)  [unwired: 9 out]
  n153 = Build Array(w138, w137) -> (w136:u32[][])
  n154 = for {
    N: w62 -> [_]
    tunnel: w259 -> [w515] mode=indexing
    shift-right: [w513] -> w128
    shift-left: w270 -> [w514]
    n155 = call "IMAQ Dispose"("All Images? (No)"=FALSE, "Image"=w515, "error in (no error)"=w514) -> ("error out"=w513:errorcluster)  [unwired: 3 out]
  }
  n156 = TDMS Write(0:w134, 5:"WhiskerCam" ("group name in (Untitled)"), 7:string[] ["BufferNumber", "BuffersDropped"] ("channel name(s) in (Untitled)"), 9:w136, 11:w135) -> (4:w132:refnum<k34>, 15:w133:errorcluster)  [unwired: 1 in, 2 out]
  n157 = TDMS Close(8:w133, 11:w132) -> (0:w131:errorcluster, 3:w116:path)
  n158 = TDMS Defragment(4:w131, 7:w116) -> (0:w112:errorcluster)
  n159 = Path To String(path=w116) -> (string=w118:string)
  n160 = Concatenate Strings(w118, "_index" ("string")) -> (w115:string)
  n161 = String To Path(string=w115) -> (path=w114:path)
  n162 = Move(source path=w126, error in=w128, 10:"Target Path") -> (error out=w127:errorcluster)  [unwired: 2 in, 2 out]
  n163 = Move(source path=w114, error in=w112, 10:"Target Path") -> ()  [unwired: 2 in, 3 out]
  n164 = Move(source path=w116, error in=w112, 10:"Target Path") -> (error out=w121:errorcluster)  [unwired: 2 in, 2 out]
  n165 = Move(source path=w123, error in=w122, 10:"Target Path") -> (error out=w120:errorcluster)  [unwired: 2 in, 2 out]
  n166 = Move(source path=w124, error in=w125, 10:"Target Path") -> (error out=w119:errorcluster)  [unwired: 2 in, 2 out]
  n167 = call <vilib>:"Simple Error Handler.vi"("error in (no error)"=w127) -> ()  [unwired: 1 in, 8 out]
  n168 = call <vilib>:"Simple Error Handler.vi"("error in (no error)"=w121) -> ()  [unwired: 1 in, 8 out]
  n169 = call <vilib>:"Simple Error Handler.vi"("error in (no error)"=w120) -> ()  [unwired: 1 in, 8 out]
  n170 = call <vilib>:"Simple Error Handler.vi"("error in (no error)"=w119) -> ()  [unwired: 1 in, 8 out]
